vi "robot movement.vi"(9 "Array 4":i32[](array[numeric]), 10 "Array 2":dbl[](array[numeric]), 11 "Array":dbl[](array[numeric])) -> (3 "Array 3":dbl[](array[numeric]))   [LabVIEW 2017]
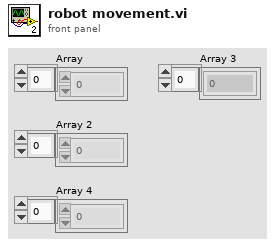
[diagram p1: front panel]
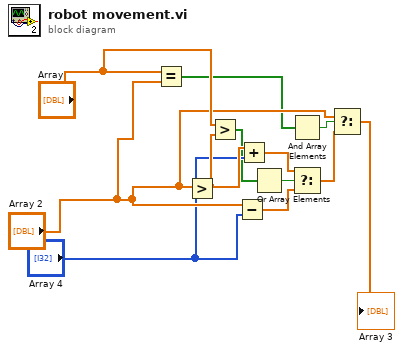
[diagram p0: block diagram]
diagram:
  n1 = Equal?(x="Array", y="Array 2") -> (x = y?=w1:bool[])
  n2 = Greater?() -> ()  [unwired: 2 in, 1 out]
  n3 = Greater?(x="Array", y="Array 2") -> (0:w3:bool[])
  n4 = Subtract(x="Array 2", y="Array 4") -> (x-y=w7:dbl[])
  n5 = Add(x="Array 2", y="Array 4") -> (x+y=w6:dbl[])
  n6 = Or Array Elements(Boolean array=w3) -> (logical OR=w4:bool)
  n7 = And Array Elements(Boolean array=w1) -> (logical AND=w2:bool)
  n8 = Select(t=w6, s=w4, f=w7) -> (s? t:f=w5:dbl[])
  n9 = Select(t="Array 2", s=w2, f=w5) -> (s? t:f=→"Array 3":dbl[])
